vi "Doe_Julabo_Control_Standalone.vi"(0 "Julabo CF41 VISA":refnum<visa-resource-name>="COM3", 1 "Data Cluster In":T1={"Current DoE"=[], "SSI 1 Flow Rate"=0.0, "SSI 2 Flow Rate"=0.0, "FLOM 1 Flow Rate"=0.0, "FLOM 2 Flow Rate"=0.0, "Pumps Running?"=FALSE, "Boolean 2"=FALSE, "Boolean 3"=FALSE, "Boolean 4"=FALSE, "At Equilibrium?"=FALSE, "Script Running?"=FALSE, "Current Script Iteration"=0.0, "Total Script Iterations"=0.0, "FLOM Pumps VISA"="COM2", "SSI 1 Pump VISA"="COM76", "SSI 2 Pump VISA"="COM74", "Huber Unistat VISA"="COM1", "SSI 3 Pump VISA"="COM76", "SSI 4 Pump VISA"="COM76", "SSI 4 Flow Rate"=0.0, "SSI 3 Flow Rate"=0.0, "Flow Meter 1 Rate "=0.0, "Flow Meter 2 Rate"=0.0, "Flow Meter 3 Rate"=0.0, "Flow Meter 4 Rate"=0.0, "SSI 1 Flow Setpoint"=0.0, "SSI 2 Flow Setpoint"=0.0, "SSI 3 Flow Setpoint"=0.0, "SSI 4 Flow Setpoint"=0.0, "Temperature Setpoint"=0.0, "Flow meter 3 COM"=17, "Flow meter 5 COM"=18, "Flow meter 4 COM"=19, "Flow meter 2 COM"=16, "Flow meter 1 COM"=15, "Unit"=enum."PSI", "Pressure COM"="COM6", "Julabo Setpoint"=0.0, "Julabo Control"=enum."Internal", "Overtemp"=50.0, "Subtemp"=-20.0, "HeatMax"=50, "CoolMax"=-100, "InternMax"=50.0, "InternMin"=0.0, "Upper Bandlimit"=100.0, "Lower Bandlimit"=0.0, "Julabo CF41 VISA"="COM3", "Xp (0.6K) Int"=0.6, "Tn (3s) Int"=3, "Tv (0s) Int"=0, "Dynamic (0: aperiodic) Int"=enum."aperiodic", "Xp (0.6K) Ext"=0.6, "Tn (3s) Ext"=3, "Tv (0s) Ext"=0, "XpU (0.6K) Ext"=0.6} {"XpU (0.6K) Ext" min=0.1 max=99.9; "Tv (0s) Ext" max=999; "Tn (3s) Ext" min=3 max=9999; "Xp (0.6K) Ext" min=0.1 max=99.9; "Tv (0s) Int" max=999; "Tn (3s) Int" min=3 max=9999; "Xp (0.6K) Int" min=0.1 max=99.9; "Lower Bandlimit" min=0.0 max=200.0; "Upper Bandlimit" min=0.0 max=200.0; "InternMin" format="%.2f"; "InternMax" format="%.2f"; "CoolMax" min=-100 max=0; "HeatMax" max=100; "Subtemp" format="%.2f"; "Overtemp" format="%.2f"; "Julabo Setpoint" format="%.2f"; "Current DoE" format="%0.3f"}, 5 "Serial Configuration":T4={"Baud Rate"=4800, "Parity"=2, "Data Bits"=7, "Stop Bits"=10, "Flow Control"=2} {"Flow Control" items=["None", "XON/XOFF", "RTS/CTS", "XON/XOFF & RTS/CTS", "DTR/DSR", "XON/XOFF & DTR/DSR"]; "Stop Bits" items=["1.0"=10, "1.5"=15, "2.0"=20]; "Data Bits" items=["7"=7, "8"=8]; "Parity" items=["None", "Odd", "Even", "Mark", "Space"]; "Baud Rate" items=["300"=300, "600"=600, "1200"=1200, "2400"=2400, "4800"=4800, "9600"=9600, "19200"=19200]}, 7 "RS485-Address (128: RS232)":u32=128, 9 "ID Query? (T: Yes)":bool=TRUE, 11 "ReadCycle":i32=1000) -> (4 "Data Cluster Out":T1={"Current DoE"=[], "SSI 1 Flow Rate"=0.0, "SSI 2 Flow Rate"=0.0, "FLOM 1 Flow Rate"=0.0, "FLOM 2 Flow Rate"=0.0, "Pumps Running?"=FALSE, "Boolean 2"=FALSE, "Boolean 3"=FALSE, "Boolean 4"=FALSE, "At Equilibrium?"=FALSE, "Script Running?"=FALSE, "Current Script Iteration"=0.0, "Total Script Iterations"=0.0, "FLOM Pumps VISA"="COM2", "SSI 1 Pump VISA"="COM76", "SSI 2 Pump VISA"="COM74", "Huber Unistat VISA"="COM1", "SSI 3 Pump VISA"="COM76", "SSI 4 Pump VISA"="COM76", "SSI 4 Flow Rate"=0.0, "SSI 3 Flow Rate"=0.0, "Flow Meter 1 Rate "=0.0, "Flow Meter 2 Rate"=0.0, "Flow Meter 3 Rate"=0.0, "Flow Meter 4 Rate"=0.0, "SSI 1 Flow Setpoint"=0.0, "SSI 2 Flow Setpoint"=0.0, "SSI 3 Flow Setpoint"=0.0, "SSI 4 Flow Setpoint"=0.0, "Temperature Setpoint"=0.0, "Flow meter 3 COM"=17, "Flow meter 5 COM"=18, "Flow meter 4 COM"=19, "Flow meter 2 COM"=16, "Flow meter 1 COM"=15, "Unit"=enum."PSI", "Pressure COM"="COM6", "Julabo Setpoint"=0.0, "Julabo Control"=enum."Internal", "Overtemp"=50.0, "Subtemp"=-20.0, "HeatMax"=50, "CoolMax"=-100, "InternMax"=50.0, "InternMin"=0.0, "Upper Bandlimit"=100.0, "Lower Bandlimit"=0.0, "Julabo CF41 VISA"="COM3", "Xp (0.6K) Int"=0.6, "Tn (3s) Int"=3, "Tv (0s) Int"=0, "Dynamic (0: aperiodic) Int"=enum."aperiodic", "Xp (0.6K) Ext"=0.6, "Tn (3s) Ext"=3, "Tv (0s) Ext"=0, "XpU (0.6K) Ext"=0.6} {"XpU (0.6K) Ext" min=0.1 max=99.9; "Tv (0s) Ext" max=999; "Tn (3s) Ext" min=3 max=9999; "Xp (0.6K) Ext" min=0.1 max=99.9; "Tv (0s) Int" max=999; "Tn (3s) Int" min=3 max=9999; "Xp (0.6K) Int" min=0.1 max=99.9; "Lower Bandlimit" min=0.0 max=200.0; "Upper Bandlimit" min=0.0 max=200.0; "InternMin" format="%.2f"; "InternMax" format="%.2f"; "CoolMax" min=-100 max=0; "HeatMax" max=100; "Subtemp" format="%.2f"; "Overtemp" format="%.2f"; "Julabo Setpoint" format="%.2f"; "Current DoE" format="%0.3f"}, 6 "Internal Temp":dbl format="%.2f", 8 "External Temp":dbl format="%.2f", 15 "device error out":errorcluster)   [LabVIEW 2015, in "JULABO DeviceDriver.lvlib"]
doc: "Advanced event triggered example"
uses:
  <instrlib>/JULABO DeviceDriver/JULABO DeviceDriver.lvlib
  <instrlib>/JULABO DeviceDriver/Examples/Julabo Serial Control.ctl
  --Controls and TypeDefs--/DoE_Control_Cluster.ctl
panel:
  out "error out 2":errorcluster caption="error out"
  out "error out":errorcluster
  in  "Registerkartenelement":T2(tab)
  out "Safety Temp":dbl
  out "Excess Temp Protection":dbl
  in  "Control":enum16{"Internal", "External"}(ring)
  in  "Setpoint":dbl format="%.2f"
  out "Power":i8(slide) scale=-100.0..100.0
  out "Diagram":T3(graph)
  in  "StartStop":bool
  in  "btnAdjustInternalTempLimits":bool
  in  "btnAdjustBandLimits":bool
  in  "btnAdjustCapacityLevels":bool
  in  "btnAdjustWarningLevels":bool
  in  "Upper Bandlimit":dbl=100.0 min=0.0 max=200.0
  in  "Lower Bandlimit":dbl min=0.0 max=200.0
  in  "InternMin":dbl format="%.2f"
  in  "InternMax":dbl=50.0 format="%.2f"
  in  "CoolMax":i8=-100 min=-100 max=0
  in  "HeatMax":u8=50 max=100
  in  "Subtemp":dbl=-20.0 format="%.2f"
  in  "Overtemp":dbl=50.0 format="%.2f"
  in  "Tv (0s) 2":u16 max=999
  in  "Tn (3s) 2":u16=3 min=3 max=9999
  in  "Xp (0.6K) 2":dbl=0.6 min=0.1 max=99.9
  in  "btnAdjustExternalControlParams":bool
  in  "XpU (0.6K)":dbl=0.6 min=0.1 max=99.9
  in  "Dynamic (0: aperiodic)":enum16{"aperiodic", "standard"}(ring)
  in  "btnAdjustInternalControlParams":bool
  in  "Tv (0s)":u16 max=999
  in  "Tn (3s)":u16=3 min=3 max=9999
  in  "Xp (0.6K)":dbl=0.6 min=0.1 max=99.9
  in  "Stopp":bool
  in  "Reset / Default (T: Both)":bool=TRUE
  # "Note: Julabo must be set to Set Temp - RS232\nfor commands to properly write to unit!!!!!"
  # "1. Select the COM-Port and adjust the serial\nconfiguration for your instrument\n2. Adjust the Read cycle\n3. Start the VI by pressing the \"Start\" -Button\n( Arrow button on the top-left corner)\n4. To stop the execution press the \"Stop\" button"
  # "Julabo"
  # "Limits"
  # "PID Control Parameters"
  # "Julabo"
  # "Limits"
  # "PID Control Parameters"
  # "Internal parameters"
  # "External parameters"
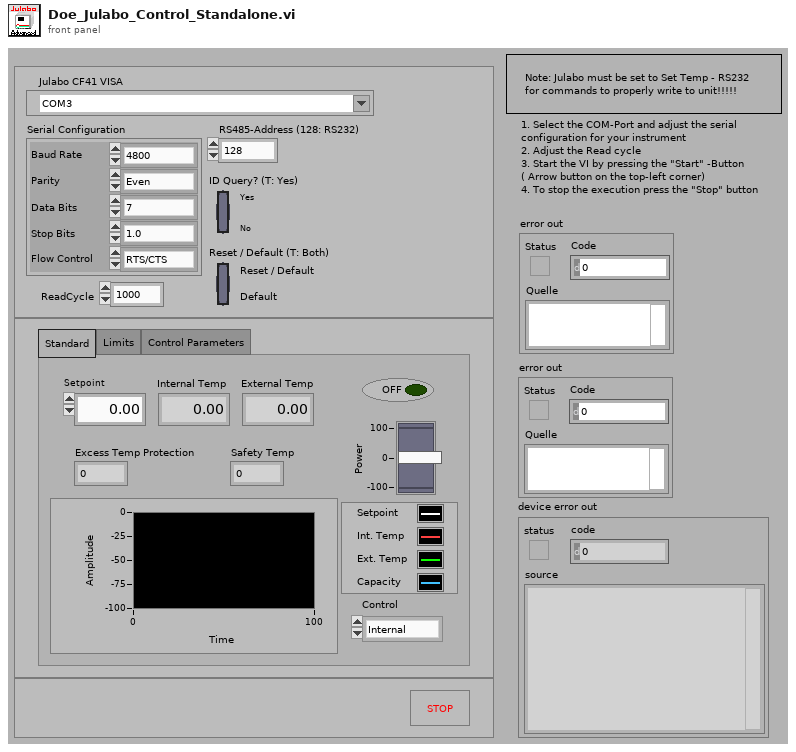
[diagram p1: front panel]
types:
  T1 = typedef "DoE_Control_Cluster.ctl" = cluster{"Current DoE":dbl[][], "SSI 1 Flow Rate":dbl, "SSI 2 Flow Rate":dbl, "FLOM 1 Flow Rate":dbl, "FLOM 2 Flow Rate":dbl, "Pumps Running?":bool, "Boolean 2":bool, "Boolean 3":bool, "Boolean 4":bool, "At Equilibrium?":bool, "Script Running?":bool, "Current Script Iteration":dbl, "Total Script Iterations":dbl, "FLOM Pumps VISA":refnum<visa-resource-name>, "SSI 1 Pump VISA":refnum<visa-resource-name>, "SSI 2 Pump VISA":refnum<visa-resource-name>, "Huber Unistat VISA":refnum<visa-resource-name>, "SSI 3 Pump VISA":refnum<visa-resource-name>, "SSI 4 Pump VISA":refnum<visa-resource-name>, "SSI 4 Flow Rate":dbl, "SSI 3 Flow Rate":dbl, "Flow Meter 1 Rate ":dbl, "Flow Meter 2 Rate":dbl, "Flow Meter 3 Rate":dbl, "Flow Meter 4 Rate":dbl, "SSI 1 Flow Setpoint":dbl, "SSI 2 Flow Setpoint":dbl, "SSI 3 Flow Setpoint":dbl, "SSI 4 Flow Setpoint":dbl, "Temperature Setpoint":dbl, "Flow meter 3 COM":u16, "Flow meter 5 COM":u16, "Flow meter 4 COM":u16, "Flow meter 2 COM":u16, "Flow meter 1 COM":u16, "Unit":enum16{"PSI", "Bar", "cm H2O", "ft H2O", "hectoPascal", "in Hg", "in H2O", "kiloPascal", "milliBar", "mmHg", "MegaPascal", "Numeric Pressure"}, "Pressure COM":refnum<visa-resource-name>, "Julabo Setpoint":dbl, "Julabo Control":enum16{"Internal", "External"}, "Overtemp":dbl, "Subtemp":dbl, "HeatMax":u8, "CoolMax":i8, "InternMax":dbl, "InternMin":dbl, "Upper Bandlimit":dbl, "Lower Bandlimit":dbl, "Julabo CF41 VISA":refnum<visa-resource-name>, "Xp (0.6K) Int":dbl, "Tn (3s) Int":u16, "Tv (0s) Int":u16, "Dynamic (0: aperiodic) Int":enum16{"aperiodic", "standard"}, "Xp (0.6K) Ext":dbl, "Tn (3s) Ext":u16, "Tv (0s) Ext":u16, "XpU (0.6K) Ext":dbl}
  T2 = enum32{"Standard", "Limits", "Control Parameters"}
  T3 = cluster{"Setpoint (out)":dbl, "InternalTemp (out)":dbl, "ExternalTemp (out)":dbl, "Capacity (out)":i8}
  T4 = typedef "Julabo Serial Control.ctl" = cluster{"Baud Rate":u32, "Parity":u16, "Data Bits":u16, "Stop Bits":u16, "Flow Control":u16}
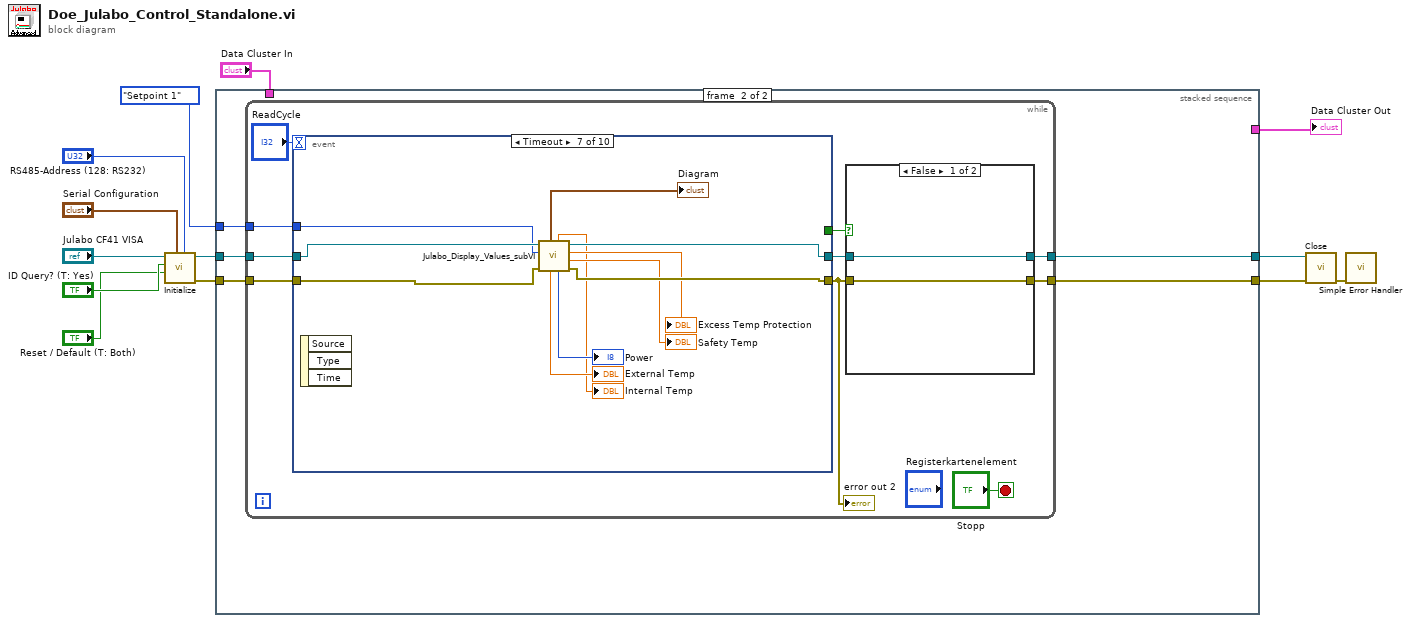
[diagram p0: block diagram]
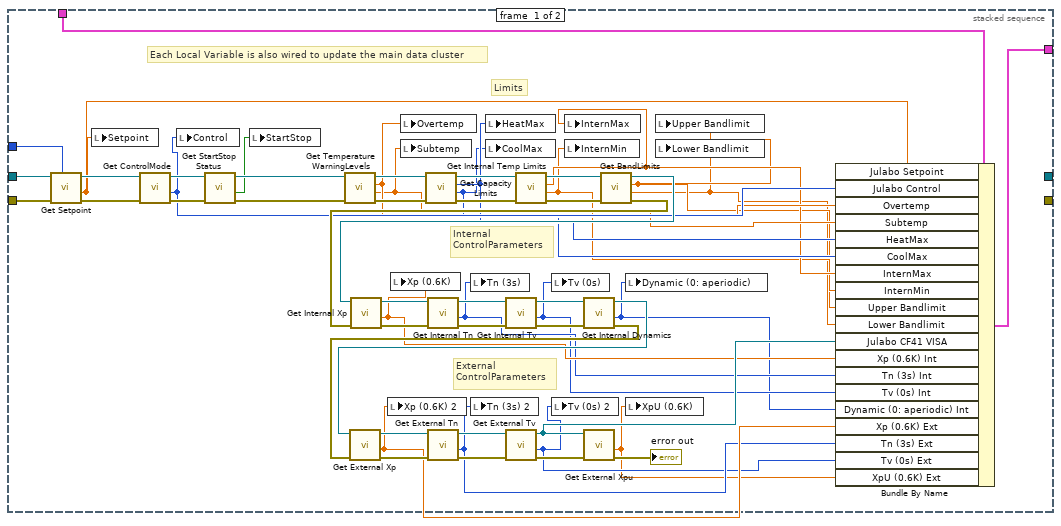
[diagram p2: hidden frame]
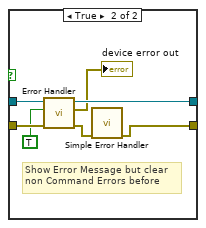
[diagram p3: hidden frame]
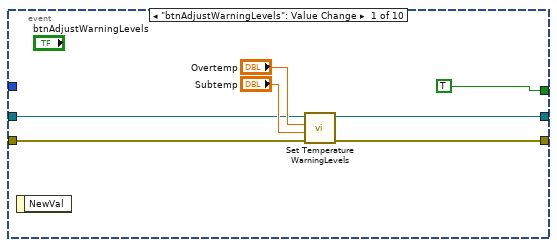
[diagram p4: hidden frame]
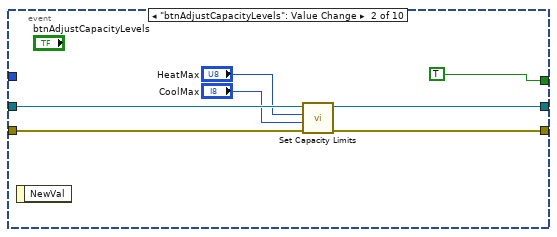
[diagram p5: hidden frame]
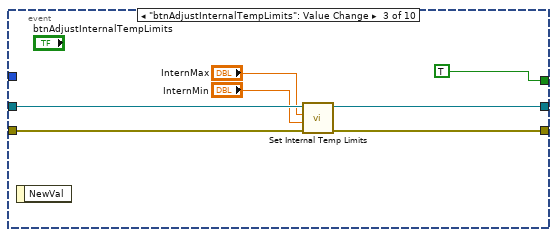
[diagram p6: hidden frame]
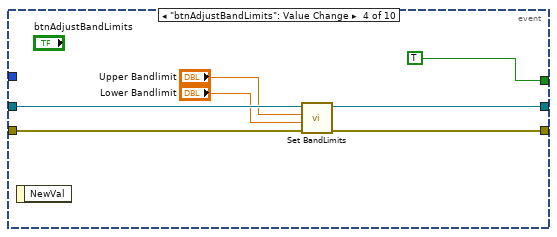
[diagram p7: hidden frame]
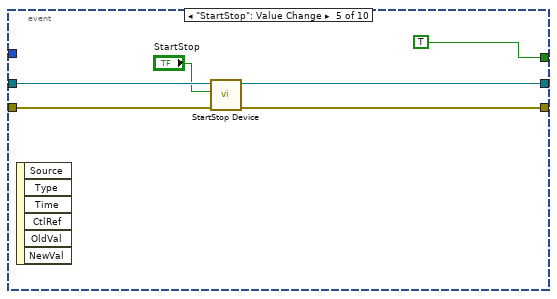
[diagram p8: hidden frame]
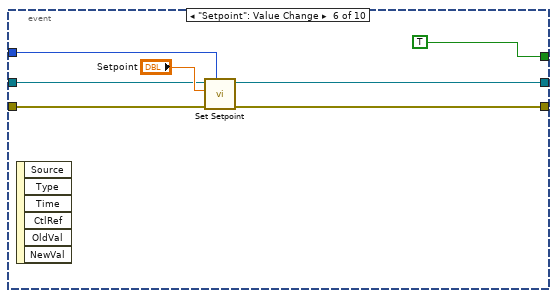
[diagram p9: hidden frame]
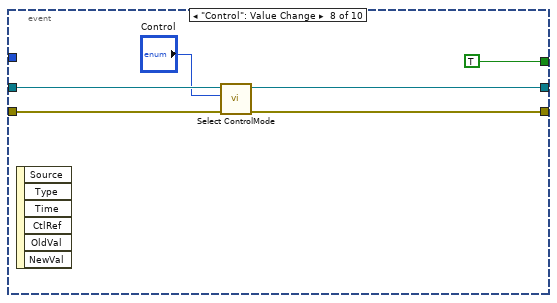
[diagram p10: hidden frame]
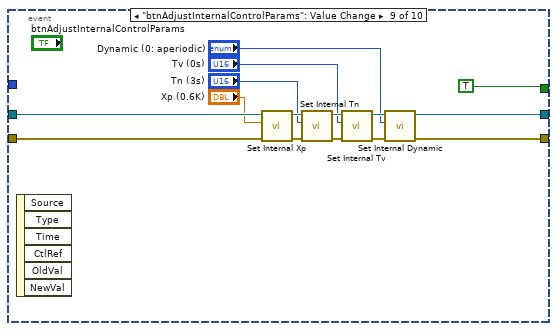
[diagram p11: hidden frame]
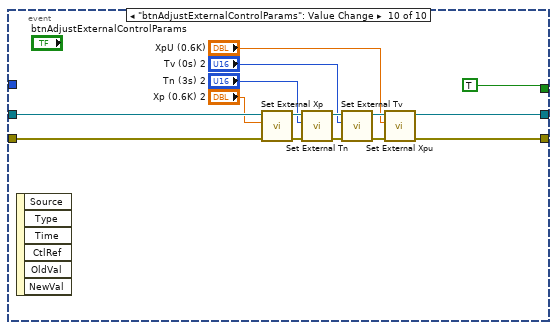
[diagram p12: hidden frame]
diagram:
  n1 = call <instrlib>:"Initialize.vi"("RS485-Address (128: RS232)"="RS485-Address (128: RS232)", "Serial Configuration"="Serial Configuration", "Reset / Default (T: Both)"="Reset / Default (T: Both)", "ID Query? (T: Yes)"="ID Query? (T: Yes)", "VISA resource name"="Julabo CF41 VISA") -> ("error out"=w6:errorcluster, "VISA resource name out"=w7:refnum<visa-resource-name>)  [unwired: 5 in]
  n2 = stacked-sequence {
    tunnel: w7 -> [w39 w71]
    tunnel: w6 -> [w38 w70]
    tunnel: [_ w69] -> w5
    tunnel: [_ w68] -> w4
    tunnel: enum16{"Setpoint 1", "Setpoint 2", "Setpoint 3"}."Setpoint 1" ("Setpointindex") -> [w35 w67]
    tunnel: "Data Cluster In" -> [w34 _]
    tunnel: [w33 _] -> w1
    frame #0 {
      # "Each Local Variable is also wired to update the main data cluster"
      # "External\nControlParameters"
      # "Internal\nControlParameters"
      # "Limits"
      n3 = call <instrlib>:"Get Setpoint.vi"("Setpointindex"=w35, "error in (no error)"=w38, "VISA resource name"=w39) -> ("error out"=w36:errorcluster, "Setpoint (out)"=w32:dbl, "VISA resource name out"=w37:refnum<visa-resource-name>)  [unwired: 6 in]
      n4 = local write "Setpoint"(w32) -> ()
      n5 = call <instrlib>:"Get ControlMode.vi"("error in"=w36, "VISA resource name in"=w37) -> ("error out"=w41:errorcluster, "Control (out)"=w31:enum16{"Internal", "External"}, "VISA resource name out"=w45:refnum<visa-resource-name>)  [unwired: 7 in]
      n6 = local write "Control"(w31) -> ()
      n7 = call <instrlib>:"Get StartStop Status.vi"("error in"=w41, "VISA resource name in"=w45) -> ("error out"=w40:errorcluster, "Status"=w42:bool, "VISA resource name out"=w43:refnum<visa-resource-name>)  [unwired: 7 in]
      n8 = local write "StartStop"(w42) -> ()
      n9 = call <instrlib>:"Get Temperature WarningLevels.vi"("error in (no error)"=w40, "VISA resource name"=w43) -> ("error out"=w63:errorcluster, "Subtemp (out)"=w29:dbl, "Overtemp (out)"=w30:dbl, "VISA resource name out"=w66:refnum<visa-resource-name>)  [unwired: 2 in]
      n10 = local write "Overtemp"(w30) -> ()
      n11 = local write "Subtemp"(w29) -> ()
      n12 = call <instrlib>:"Get Capacity Limits.vi"("error in (no error)"=w63, "VISA resource name"=w66) -> ("error out"=w62:errorcluster, "Maximum cooling capacity(out)"=w27:i8, "Maximum heating capacity(out)"=w28:u8, "VISA resource name out"=w65:refnum<visa-resource-name>)  [unwired: 2 in]
      n13 = local write "HeatMax"(w28) -> ()
      n14 = local write "CoolMax"(w27) -> ()
      n15 = call <instrlib>:"Get Internal Temp Limits.vi"("error in (no error)"=w62, "VISA resource name"=w65) -> ("error out"=w61:errorcluster, "IntMin (out)"=w25:dbl, "IntMax (out)"=w26:dbl, "VISA resource name out"=w64:refnum<visa-resource-name>)  [unwired: 2 in]
      n16 = local write "InternMax"(w26) -> ()
      n17 = local write "InternMin"(w25) -> ()
      n18 = call <instrlib>:"Get BandLimits.vi"("error in (no error)"=w61, "VISA resource name"=w64) -> ("error out"=w53:errorcluster, "LowerBand (out)"=w23:dbl, "UpperBand (out)"=w24:dbl, "VISA resource name out"=w54:refnum<visa-resource-name>)  [unwired: 2 in]
      n19 = call <instrlib>:"Get Internal Xp.vi"("error in"=w53, "VISA resource name in"=w54) -> ("error out"=w55:errorcluster, "InternalXp (out)"=w21:dbl, "VISA resource name out"=w56:refnum<visa-resource-name>)  [unwired: 7 in]
      n20 = local write "Xp (0.6K)"(w21) -> ()
      n21 = call <instrlib>:"Get Internal Tn.vi"("error in"=w55, "VISA resource name in"=w56) -> ("error out"=w57:errorcluster, "InternalTn (out)"=w20:u16, "VISA resource name out"=w58:refnum<visa-resource-name>)  [unwired: 7 in]
      n22 = local write "Tn (3s)"(w20) -> ()
      n23 = call <instrlib>:"Get Internal Tv.vi"("error in"=w57, "VISA resource name in"=w58) -> ("error out"=w59:errorcluster, "InternalTv (out)"=w19:u16, "VISA resource name out"=w60:refnum<visa-resource-name>)  [unwired: 7 in]
      n24 = local write "Tv (0s)"(w19) -> ()
      n25 = call <instrlib>:"Get Internal Dynamics.vi"("error in"=w59, "VISA resource name in"=w60) -> ("error out"=w48:errorcluster, "Dynamic (out)"=w18:enum16{"aperiodic", "standard"}, "VISA resource name out"=w47:refnum<visa-resource-name>)  [unwired: 7 in]
      n26 = call <instrlib>:"Get External Xp.vi"("error in"=w48, "VISA resource name in"=w47) -> ("error out"=w49:errorcluster, "ExternalXp (out)"=w17:dbl, "VISA resource name out"=w46:refnum<visa-resource-name>)  [unwired: 7 in]
      n27 = local write "Xp (0.6K) 2"(w17) -> ()
      n28 = call <instrlib>:"Get External Tn.vi"("error in"=w49, "VISA resource name in"=w46) -> ("error out"=w52:errorcluster, "ExternalTn (out)"=w16:u16, "VISA resource name out"=w51:refnum<visa-resource-name>)  [unwired: 7 in]
      n29 = local write "Tn (3s) 2"(w16) -> ()
      n30 = call <instrlib>:"Get External Tv.vi"("error in"=w52, "VISA resource name in"=w51) -> ("error out"=w50:errorcluster, "ExternalTv (out)"=w15:u16, "VISA resource name out"=w22:refnum<visa-resource-name>)  [unwired: 7 in]
      n31 = local write "Tv (0s) 2"(w15) -> ()
      n32 = call <instrlib>:"Get External Xpu.vi"("error in"=w50, "VISA resource name in"=w22) -> ("error out"=→"error out":errorcluster, "ExternalXpu (out)"=w14:dbl)  [unwired: 7 in, 1 out]
      n33 = local write "Dynamic (0: aperiodic)"(w18) -> ()
      n34 = local write "XpU (0.6K)"(w14) -> ()
      n35 = local write "Upper Bandlimit"(w24) -> ()
      n36 = local write "Lower Bandlimit"(w23) -> ()
      n37 = Bundle By Name(cluster=w34, "Julabo Setpoint"=w32, "Julabo Control"=w31, "Overtemp"=w30, "Subtemp"=w29, "HeatMax"=w28, "CoolMax"=w27, "InternMax"=w26, "InternMin"=w25, "Upper Bandlimit"=w24, "Lower Bandlimit"=w23, "Julabo CF41 VISA"=w22, "Xp (0.6K) Int"=w21, "Tn (3s) Int"=w20, "Tv (0s) Int"=w19, "Dynamic (0: aperiodic) Int"=w18, "Xp (0.6K) Ext"=w17, "Tn (3s) Ext"=w16, "Tv (0s) Ext"=w15, "XpU (0.6K) Ext"=w14) -> (w33:T1)
    }
    frame #1 {
      n38 = while {
        tunnel: w71 -> [w81]
        tunnel: w70 -> [w80]
        tunnel: [w78] -> w68
        tunnel: [w77] -> w69
        tunnel: w67 -> [w73]
        stop <- "Stopp" stop-if-true
        n39 = event shown="[6] Timeout" {
          selector: _ -> [_ _ _ _ _ _ _ _ _ _]
          dyn-events: _ -> [_ _ _ _ _ _ _ _ _ _]
          timeout: "ReadCycle" -> [_ _ _ _ _ _ _ _ _ _]
          tunnel: [w92 w100 w110 w117 w121 w128 w140 w146 w152 w167] -> w79
          tunnel: [w91 w99 w109 w116 w122 w127 w139 w145 w150 w165] -> w72
          tunnel: w81 -> [w95 w104 w108 w114 w120 w130 w142 w148 w163 w178]
          tunnel: w80 -> [w94 w103 w107 w115 w123 w129 w141 w147 w162 w177]
          tunnel: [TRUE TRUE TRUE TRUE TRUE TRUE _ TRUE TRUE TRUE] -> w76
          tunnel: w73 -> [_ _ _ _ _ w125 w138 _ _ _]
          event "btnAdjustWarningLevels": Value Change {
            n40 = event-data() -> ()  [unwired: 1 in, 1 out]
            n41 = call <instrlib>:"Set Temperature WarningLevels.vi"("error in (no error)"=w94, "Subtemp (-20.00°C)"="Subtemp", "Overtemp (50.00°C)"="Overtemp", "VISA resource name"=w95) -> ("error out"=w91:errorcluster, "VISA resource name out"=w92:refnum<visa-resource-name>)  [unwired: 6 in]
          }
          event "btnAdjustCapacityLevels": Value Change {
            n42 = event-data() -> ()  [unwired: 1 in, 1 out]
            n43 = call <instrlib>:"Set Capacity Limits.vi"("error in (no error)"=w103, "Maximum cooling capacity(-100%)"="CoolMax", "Maximum heating capacity(100%)"="HeatMax", "VISA resource name"=w104) -> ("error out"=w99:errorcluster, "VISA resource name out"=w100:refnum<visa-resource-name>)  [unwired: 6 in]
          }
          event "btnAdjustInternalTempLimits": Value Change {
            n44 = event-data() -> ()  [unwired: 1 in, 1 out]
            n45 = call <instrlib>:"Set Internal Temp Limits.vi"("error in (no error)"=w107, "InternMin (-20.00 °C)"="InternMin", "InternMax (50.00 °C)"="InternMax", "VISA resource name"=w108) -> ("error out"=w109:errorcluster, "VISA resource name out"=w110:refnum<visa-resource-name>)  [unwired: 6 in]
          }
          event "btnAdjustBandLimits": Value Change {
            n46 = event-data() -> ()  [unwired: 1 in, 1 out]
            n47 = call <instrlib>:"Set BandLimits.vi"("error in (no error)"=w115, "Lower Bandlimit (200K)"="Lower Bandlimit", "Upper Bandlimit (200K)"="Upper Bandlimit", "VISA resource name"=w114) -> ("error out"=w116:errorcluster, "VISA resource name out"=w117:refnum<visa-resource-name>)  [unwired: 6 in]
          }
          event "StartStop": Value Change {
            n48 = event-data() -> ()  [unwired: 1 in, 6 out]
            n49 = call <instrlib>:"StartStop Device.vi"("error in (no error)"=w123, "Start/Stop (f:Stop)"="StartStop", "VISA resource name"=w120) -> ("error out"=w122:errorcluster, "VISA resource name out"=w121:refnum<visa-resource-name>)  [unwired: 7 in]
          }
          event "Setpoint": Value Change {
            n50 = event-data() -> ()  [unwired: 1 in, 6 out]
            n51 = call <instrlib>:"Set Setpoint.vi"("Setpointindex (Setpoint1: Default)"=w125, "error in (no error)"=w129, "newSetpoint (20.00°C)"="Setpoint", "VISA resource name"=w130) -> ("error out"=w127:errorcluster, "VISA resource name out"=w128:refnum<visa-resource-name>)  [unwired: 6 in]
          }
          event Timeout {
            n52 = event-data() -> ()  [unwired: 1 in, 3 out]
            n53 = call "Julabo_Display_Values_subVI.vi"("error in (no error)"=w141, "Setpointindex"=w138, "VISA Refnum in"=w142) -> ("error out"=w139:errorcluster, "Safety Temp"=→"Safety Temp":dbl, "Excess Temp Protection"=→"Excess Temp Protection":dbl, "VISA Refnum out"=w140:refnum<visa-resource-name>, "Power"=→"Power":i8, "Internal Temp"=→"Internal Temp":dbl, "External Temp"=→"External Temp":dbl, "Diagram"=→"Diagram":T3)  [unwired: 1 in]
          }
          event "Control": Value Change {
            n54 = event-data() -> ()  [unwired: 1 in, 6 out]
            n55 = call <instrlib>:"Select ControlMode.vi"("error in (no error)"=w147, "Control (0: Internal)"="Control", "VISA resource name"=w148) -> ("error out"=w145:errorcluster, "VISA resource name out"=w146:refnum<visa-resource-name>)  [unwired: 7 in]
          }
          event "btnAdjustInternalControlParams": Value Change {
            n56 = event-data() -> ()  [unwired: 1 in, 6 out]
            n57 = call <instrlib>:"Set Internal Xp.vi"("error in (no error)"=w162, "Xp (0.6K)"="Xp (0.6K)", "VISA resource name"=w163) -> ("error out"=w159:errorcluster, "VISA resource name out"=w158:refnum<visa-resource-name>)  [unwired: 7 in]
            n58 = call <instrlib>:"Set Internal Tn.vi"("error in (no error)"=w159, "Tn (3s)"="Tn (3s)", "VISA resource name"=w158) -> ("error out"=w161:errorcluster, "VISA resource name out"=w160:refnum<visa-resource-name>)  [unwired: 7 in]
            n59 = call <instrlib>:"Set Internal Tv.vi"("error in (no error)"=w161, "Tv (0s)"="Tv (0s)", "VISA resource name"=w160) -> ("error out"=w151:errorcluster, "VISA resource name out"=w154:refnum<visa-resource-name>)  [unwired: 7 in]
            n60 = call <instrlib>:"Set Internal Dynamic.vi"("error in (no error)"=w151, "Dynamic (0: aperiodic)"="Dynamic (0: aperiodic)", "VISA resource name"=w154) -> ("error out"=w150:errorcluster, "VISA resource name out"=w152:refnum<visa-resource-name>)  [unwired: 7 in]
          }
          event "btnAdjustExternalControlParams": Value Change {
            n61 = event-data() -> ()  [unwired: 1 in, 6 out]
            n62 = call <instrlib>:"Set External Xp.vi"("error in (no error)"=w177, "Xp (0.6K)"="Xp (0.6K) 2", "VISA resource name"=w178) -> ("error out"=w174:errorcluster, "VISA resource name out"=w173:refnum<visa-resource-name>)  [unwired: 7 in]
            n63 = call <instrlib>:"Set External Tn.vi"("error in (no error)"=w174, "Tn (3s)"="Tn (3s) 2", "VISA resource name"=w173) -> ("error out"=w176:errorcluster, "VISA resource name out"=w175:refnum<visa-resource-name>)  [unwired: 7 in]
            n64 = call <instrlib>:"Set External Tv.vi"("error in (no error)"=w176, "Tv (0s)"="Tv (0s) 2", "VISA resource name"=w175) -> ("error out"=w166:errorcluster, "VISA resource name out"=w169:refnum<visa-resource-name>)  [unwired: 7 in]
            n65 = call <instrlib>:"Set External Xpu.vi"("error in (no error)"=w166, "XpU (0.6K)"="XpU (0.6K)", "VISA resource name"=w169) -> ("error out"=w165:errorcluster, "VISA resource name out"=w167:refnum<visa-resource-name>)  [unwired: 7 in]
          }
        }
        "error out 2" <- w72
        n66 = case shown="False" w76 {
          tunnel: w79 -> [w83 w88]
          tunnel: [w83 w86] -> w78
          tunnel: w72 -> [w82 w89]
          tunnel: [w82 w90] -> w77
          frame False {
          }
          frame True {
            # "Show Error Message but clear\nnon Command Errors before"
            n67 = call <instrlib>:"Error Handler.vi"("error in (no error)"=w89, "ClearDeviceError (false)"=TRUE, "VISA resource name"=w88) -> ("error out"=w87:errorcluster, "device error out"=→"device error out":errorcluster, "VISA resource name out"=w86:refnum<visa-resource-name>)  [unwired: 5 in, 1 out]
            n68 = call <vilib>:"Simple Error Handler.vi"("error in (no error)"=w87) -> ("error out"=w90:errorcluster)  [unwired: 4 in, 4 out]
          }
        }
      }
    }
  }
  "Data Cluster Out" <- w1
  n69 = call <instrlib>:"Close.vi"("error in (no error)"=w5, "VISA resource name"=w4) -> ("error out"=w11:errorcluster)  [unwired: 9 in]
  n70 = call <vilib>:"Simple Error Handler.vi"("error in (no error)"=w11) -> ()  [unwired: 4 in, 5 out]
